vi "L_Cal_Timestamp.vi"(11 "data":u8[](array[numeric])) -> (3 "Timestamp":ext)   [LabVIEW 2019]
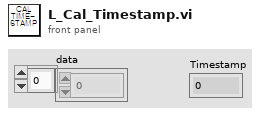
[diagram p1: front panel]
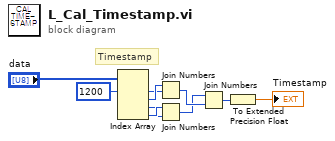
[diagram p0: block diagram]
diagram:
  # "Timestamp"
  n1 = Index Array(array="data", index #1=1200 ("index")) -> (element #1=w6:u8, element #2=w7:u8, element #3=w8:u8, element #4=w9:u8)  [unwired: 3 in]
  n2 = Join Numbers(hi=w7, lo=w6) -> ((hi.lo)=w5:u16)
  n3 = Join Numbers(hi=w9, lo=w8) -> ((hi.lo)=w4:u16)
  n4 = Join Numbers(hi=w4, lo=w5) -> ((hi.lo)=w3:u32)
  n5 = To Extended Precision Float(1:w3) -> (0:→"Timestamp":ext)
